vi "Calc dw.vi"(9 "Width T in incheees":dbl, 10 "Target":T1) -> (2 "dw":dbl)   [LabVIEW 2016]
panel:
  in  "Theta FOV":i32=67
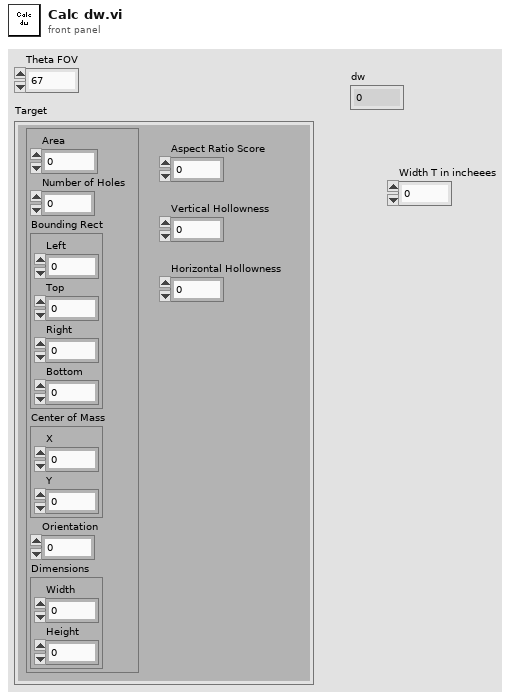
[diagram p1: front panel]
types:
  T1 = cluster{"Particle Report":cluster{"Area":dbl, "Number of Holes":dbl, "Bounding Rect":cluster{"Left":dbl, "Top":dbl, "Right":dbl, "Bottom":dbl}, "Center of Mass":cluster{"X":dbl, "Y":dbl}, "Orientation":dbl, "Dimensions":cluster{"Width":dbl, "Height":dbl}}, "Aspect Ratio Score":dbl, "Vertical Hollowness":dbl, "Horizontal Hollowness":dbl}
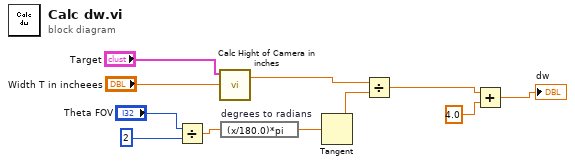
[diagram p0: block diagram]
diagram:
  n1 = Divide(x="Theta FOV", y=2) -> (x/y=w7:dbl)
  n2 = call "Calc Hight of Camera in inches.vi"("Target"="Target", "width of T in inches"="Width T in incheees") -> ("Width in inches"=w2:dbl)  [unwired: 8 in]
  n3 = expression code="(x/180.0)*pi" "degrees to radians"(w7) -> (w6:dbl)
  n4 = Tangent(1:w6) -> (0:w8:dbl)
  n5 = Divide(x=w2, y=w8) -> (x/y=w1:dbl)
  n6 = Add(x=w1, y=4.0) -> (x+y=→"dw":dbl)
